vi "go to first element.vi"(8 "error in (no error)":errorcluster, 11 "Array in":refnum<vi>) -> (0 "error out":errorcluster, 3 "reference out":refnum<vi>)   [LabVIEW 2014, in "Tagbus PID Module editor node.lvclass"]
uses:
  Tagbus PID Module editor node.lvclass
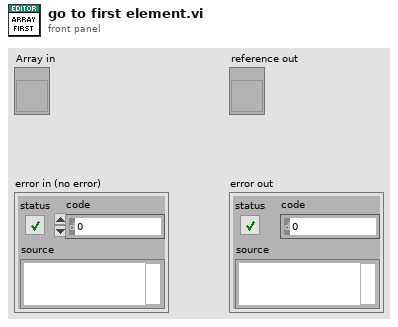
[diagram p1: front panel]
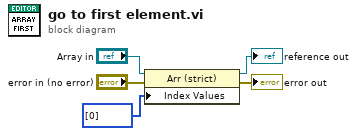
[diagram p0: block diagram]
diagram:
  n1 = property class="Arr (strict)"(reference="Array in", error in="error in (no error)", "Index Values"=u32[] [0]) -> (reference out=→"reference out":refnum<vi>, error out=→"error out":errorcluster)
